vi "Lab12Heater - Copy.vi"() -> ()   [LabVIEW 2014]
panel:
  in  "Current":dbl
  in  "Coldfinger Temp":dbl
  in  "Low Setpoint":dbl=30.0
  in  "Hi Setpoint":dbl=33.0
  in  "dt (seconds)":dbl=0.5 format="%#_13g"
  out "Sample Temp":dbl
  out "Waveform Chart":dbl(graph)
  in  "?":bool
  out "Heater Output":dbl(slide) scale=0.0..1.0
  in  "Heater Current":u16(ring) items=["Zero heat", "Low", "Medium", "High"]
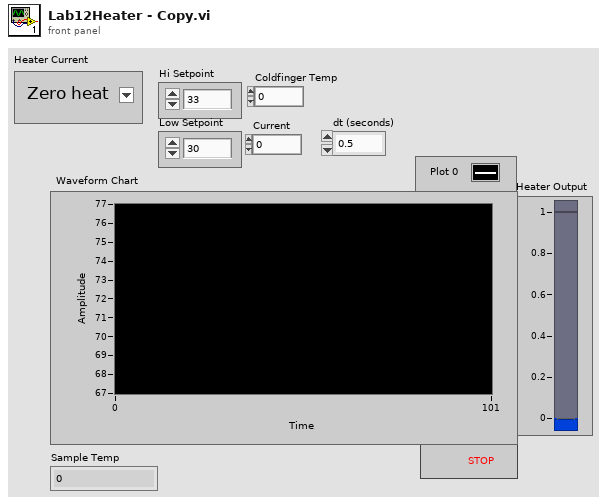
[diagram p1: front panel]
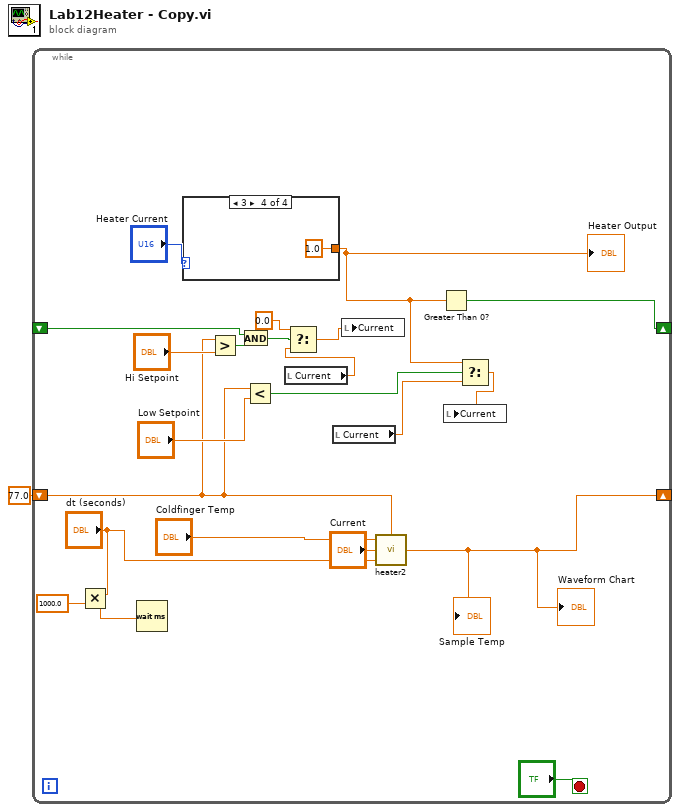
[diagram p0: block diagram]
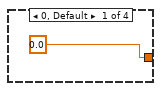
[diagram p2: hidden frame]
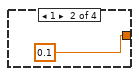
[diagram p3: hidden frame]
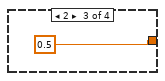
[diagram p4: hidden frame]
diagram:
  n1 = while {
    shift-right: [w22] -> _
    shift-left: 77.0 ("Tout") -> [w12]
    shift-right: [w20] -> _
    shift-left: _ -> [w9]
    stop <- "?" stop-if-true
    n2 = Multiply(x="dt (seconds)", y=1000.0) -> (x*y=w2:dbl)
    n3 = Wait (ms)(milliseconds to wait=w2) -> ()  [unwired: 1 out]
    n4 = case shown="3" "Heater Current" {
      tunnel: [0.0 0.1 0.5 1.0] -> w17
      frame 0, Default {
      }
      frame 1 {
      }
      frame 2 {
      }
      frame 3 {
      }
    }
    "Heater Output" <- w17
    n5 = Greater?(x=w12, y="Hi Setpoint") -> (0:w10:bool)
    n6 = And(x=w9, y=w10) -> (x .and. y?=w8:bool)
    n7 = Less?(x=w12, y="Low Setpoint") -> (x < y?=w15:bool)
    n8 = local read "Current"() -> (w6:dbl)
    n9 = Select(t=0.0, s=w8, f=w6) -> (s? t:f=w5:dbl)
    n10 = local read "Current"() -> (w14:dbl)
    n11 = local write "Current"(w5) -> ()
    n12 = call "heater2.vi"("Tin"=w12, "dt (seconds)"="dt (seconds)", "Current"="Current", "Tamb"="Coldfinger Temp") -> ("Tout"=w22:dbl)
    "Waveform Chart" <- w22
    "Sample Temp" <- w22
    n13 = Greater Than 0?(x=w17) -> (x > 0?=w20:bool)
    n14 = Select(t=w17, s=w15, f=w14) -> (s? t:f=w11:dbl)
    n15 = local write "Current"(w11) -> ()
  }
